vi "GenerateErrorControl.vi"(0 "VI Ref In":refnum<vi>, 5 "Label":string, 9 "Change To Indicator?":bool, 11 "Error In":errorcluster, 12 "FP Position":T1) -> (15 "Error Out":errorcluster)   [LabVIEW 2019, in "JsonToCluster.lvlib"]
doc: "This VI creates error Indicator if Change to Indicator is true, if false it cretaes error control"
uses:
  JsonToCluster.lvlib
  <vilib>/Utility/miscctls.llb/LVPositionTypeDef.ctl
  <vilib>/numeric/LVNumericRepresentation.ctl
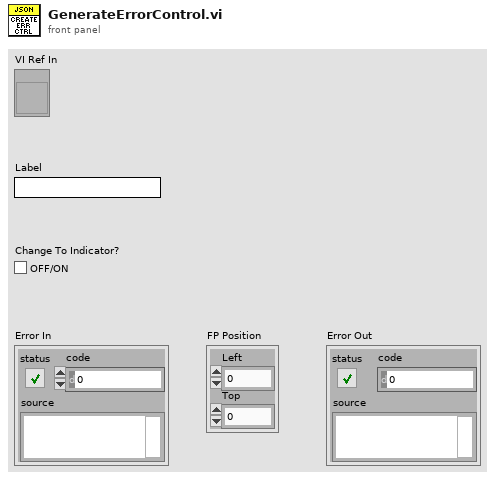
[diagram p1: front panel]
types:
  T1 = typedef "LVPositionTypeDef.ctl" = cluster{"Left":i32, "Top":i32}
  T2 = typedef "LVNumericRepresentation.ctl" = enum32{"Extended Precision", "Double Precision", "Single Precision", "Long", "Word", "Byte", "Unsigned Long", "Unsigned Word", "Unsigned Byte", "Complex Extended", "Complex Double", "Complex Single", "Quad", "Unsigned Quad", "Fixed-Point"}
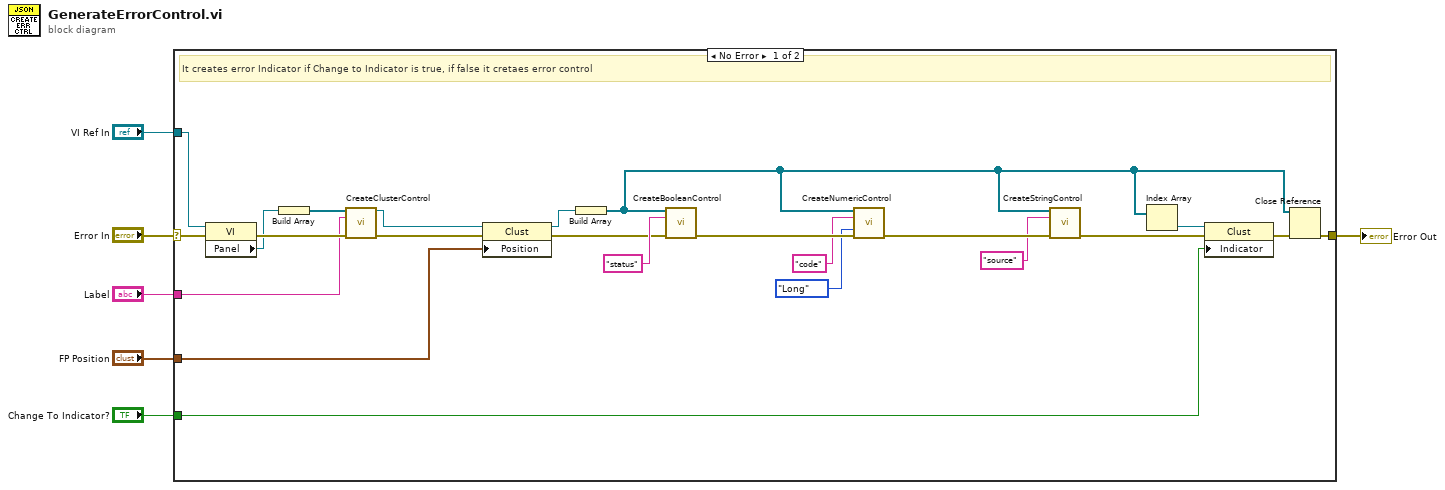
[diagram p0: block diagram]
diagram:
  n1 = case shown="No Error" "Error In" {
    selector: "Error In" -> [w23 w30]
    tunnel: [w13 w30] -> w6
    tunnel: "VI Ref In" -> [w21 _]
    tunnel: "FP Position" -> [w14 _]
    tunnel: "Change To Indicator?" -> [w7 _]
    tunnel: "Label" -> [w12 _]
    frame No Error {
      # "It creates error Indicator if Change to Indicator is true, if false it cretaes error control"
      n2 = property class="VI"(reference=w21, error in=w23) -> (error out=w22:errorcluster, "Panel"=w20:refnum<vi>)  [unwired: 1 out]
      n3 = Build Array(w20) -> (w19:refnum<vi>[])
      n4 = call "CreateClusterControl.vi"("Parent Ref In"=w19, "Cluster Label"=w12, "Error In"=w22) -> ("Cluster Ref Out"=w16:refnum<vi>, "Error Out"=w18:errorcluster)  [unwired: 11 in]
      n5 = property class="Clust"(reference=w16, error in=w18, "Position"=w14) -> (reference out=w15:refnum<vi>, error out=w17:errorcluster)
      n6 = Build Array(w15) -> (w9:refnum<vi>[])
      n7 = call "CreateBooleanControl.vi"("Parent Ref In"=w9, "Boolean Label"="status", "Error In"=w17) -> ("Error Out"=w29:errorcluster)  [unwired: 12 in]
      n8 = call "CreateNumericControl.vi"("Parent Ref In"=w9, "Control Label"="code", "Representation"=LVNumericRepresentation."Long", "Error In"=w29) -> ("Error Out"=w25:errorcluster)  [unwired: 11 in]
      n9 = call "CreateStringControl.vi"("Parent Ref In"=w9, "String Control label"="source", "Error In"=w25) -> ("Error Out"=w11:errorcluster)  [unwired: 12 in]
      n10 = Index Array(array=w9) -> (element=w8:refnum<vi>)  [unwired: 1 in]
      n11 = property class="Clust"(reference=w8, error in=w11, "Indicator"=w7) -> (error out=w10:errorcluster)  [unwired: 1 out]
      n12 = Close Reference(reference=w9, error in (no error)=w10) -> (error out=w13:errorcluster)
    }
    frame Error {
      # "If error, this case pass that error message only"
    }
  }
  "Error Out" <- w6
